vi "IsRefnum.vi"(8 "error in":errorcluster, 11 "OperationCycle in":refnum<class "OperationCycle.lvclass">) -> (0 "error out":errorcluster, 2 "IsRefnum":bool, 3 "OperationCycle out":refnum<class "OperationCycle.lvclass">)   [LabVIEW 2021, in "ProligentXMLGenerator.lvlib" / "OperationCycle.lvclass"]
doc: "Returns TRUE if the passed object is valid."
uses:
  OperationCycle.lvclass
  OperationCycle.lvclass/OperationCycle.ctl
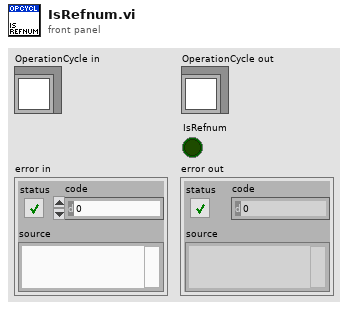
[diagram p1: front panel]
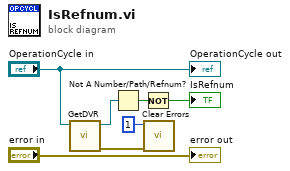
[diagram p0: block diagram]
diagram:
  n1 = call "GetDVR.vi"("OperationCycle in"="OperationCycle in") -> ("error out"=w1:errorcluster, "DVRReference"=w4:refnum<data-value>)  [unwired: 9 in]
  n2 = Not A Number/Path/Refnum?(number/path/refnum=w4) -> (NaN/Path/Refnum?=w5:bool)
  n3 = Not(x=w5) -> (.not. x?=→"IsRefnum":bool)
  n4 = call <vilib>:"Clear Errors.vi"("error in (no error)"=w1, "specific error code to clear (0: all)"=1) -> ()  [unwired: 4 in, 2 out]
  "error out" <- "error in"
  "OperationCycle out" <- "OperationCycle in"
